vi "Initialize SP.vi"(8 "error in (no error)":errorcluster, 11 "Settings in":refnum<class "Settings.lvclass">) -> (0 "error out":errorcluster, 3 "Settings out":refnum<class "Settings.lvclass">)   [LabVIEW 2023, in "GUI.lvlib" / "Settings.lvlib" / "Settings.lvclass"]
uses:
  Settings.lvclass
  HardwareAbstractionLayer_LVOOP/Database/SQL Public VI/Control/DB Options.ctl
  Settings.lvclass/Settings.ctl
  Reused Code/Subpanels Actor/subpanels/subpanel/subpanel (abstract).lvclass
  HardwareAbstractionLayer_LVOOP/Database/Database.lvclass
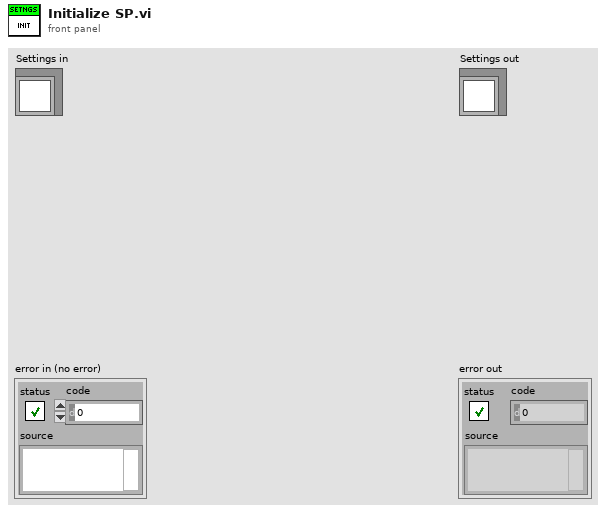
[diagram p1: front panel]
types:
  T1 = typedef "HardwareAbstractionLayer_LVOOP.lvlib/Database.lvclass/DB Options.ctl" = enum16{"Init", "Select Data", "Insert Data", "Update Data", "Delete Data", "Execute Query", "Create Schema", "Create Table", "List Tables", "List Columns", "Close"}
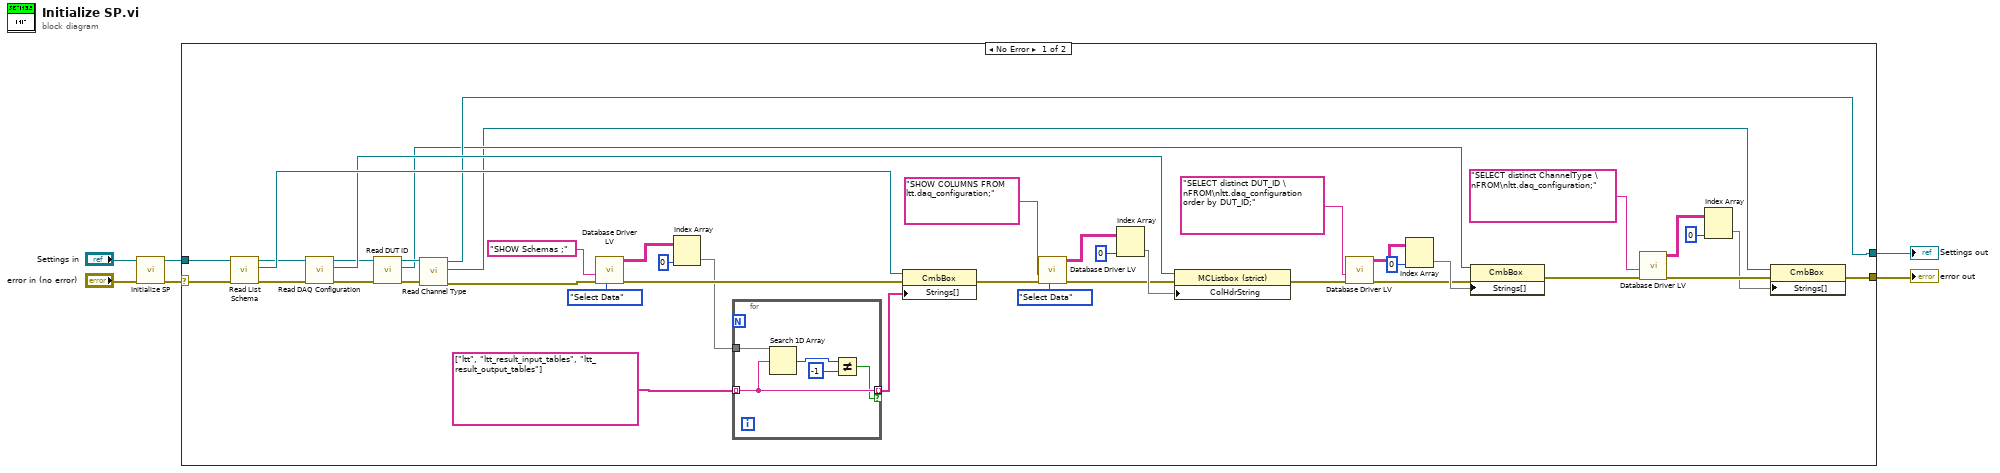
[diagram p0: block diagram]
diagram:
  n1 = call-parent "Initialize SP.vi"("error in (no error)"="error in (no error)", "subpanel (abstract) in"="Settings in") -> ("error out"=w3:errorcluster, "subpanel (abstract) out"=w4:refnum<class "Settings.lvclass">)  [unwired: 8 in]
  n2 = case shown="No Error" w3 {
    selector: w3 -> [w42 w55]
    tunnel: [w19 w55] -> w1
    tunnel: [w12 w54] -> w2
    tunnel: w4 -> [w43 w54]
    frame No Error {
      n3 = call "Read List Schema.vi"("error in (no error)"=w42, "Settings in"=w43) -> ("error out"=w33:errorcluster, "List Schema"=w41:refnum<vi>, "Settings out"=w34:refnum<class "Settings.lvclass">)  [unwired: 7 in]
      n4 = call "Read DAQ Configuration .vi"("error in (no error)"=w33, "Settings in"=w34) -> ("error out"=w17:errorcluster, "DAQ Configuration"=w32:refnum<vi>, "Settings out"=w14:refnum<class "Settings.lvclass">)  [unwired: 7 in]
      n5 = call "Read DUT ID.vi"("error in (no error)"=w17, "Settings in"=w14) -> ("error out"=w16:errorcluster, "DUT ID"=w11:refnum<vi>, "Settings out"=w13:refnum<class "Settings.lvclass">)  [unwired: 7 in]
      n6 = call "Read Channel Type.vi"("error in (no error)"=w16, "Settings in"=w13) -> ("error out"=w15:errorcluster, "Channel Type"=w10:refnum<vi>, "Settings out"=w12:refnum<class "Settings.lvclass">)  [unwired: 7 in]
      n7 = call "Database Driver LV.vi"("Options"=DB_Options."Select Data", "error in"=w15, "SQL query"="SHOW Schemas ;") -> ("error out"=w44:errorcluster, "data"=w46:string[][])  [unwired: 5 in, 2 out]
      n8 = Index Array(array=w46, index (col)=0 ("disabled index (col)")) -> (element=w8:string[])  [unwired: 1 in]
      n9 = for {
        tunnel: string[] ["ltt", "ltt_result_input_tables", "ltt_result_output_tables"] -> [w50] mode=indexing
        tunnel: w8 -> [w51]
        tunnel: [w50] -> w7 mode=indexing if=w49
        n10 = Search 1D Array(1D array=w51, element=w50) -> (index of element=w53:i32)  [unwired: 1 in]
        n11 = Not Equal?(x=w53, y=-1) -> (x != y?=w49:bool)
      }
      n12 = property on="Property Node" class="CmbBox"(reference=w41, error in=w44, "Strings[]"=w7) -> (error out=w35:errorcluster)  [unwired: 1 out]
      n13 = call "Database Driver LV.vi"("Options"=DB_Options."Select Data", "error in"=w35, "SQL query"="SHOW COLUMNS FROM ltt.daq_configuration;") -> ("error out"=w36:errorcluster, "data"=w39:string[][])  [unwired: 5 in, 2 out]
      n14 = Index Array(array=w39, index (col)=0 ("disabled index (col)")) -> (element=w37:string[])  [unwired: 1 in]
      n15 = property on="Property Node" class="MCListbox (strict)"(reference=w32, error in=w36, "ColHdrString"=w37) -> (error out=w25:errorcluster)  [unwired: 1 out]
      n16 = call "Database Driver LV.vi"("error in"=w25, "SQL query"="SELECT distinct DUT_ID \nFROM\nltt.daq_configuration order by DUT_ID;") -> ("error out"=w28:errorcluster, "data"=w30:string[][])  [unwired: 6 in, 2 out]
      n17 = Index Array(array=w30, index (col)=0 ("disabled index (col)")) -> (element=w29:string[])  [unwired: 1 in]
      n18 = property on="Property Node" class="CmbBox"(reference=w11, error in=w28, "Strings[]"=w29) -> (error out=w18:errorcluster)  [unwired: 1 out]
      n19 = call "Database Driver LV.vi"("error in"=w18, "SQL query"="SELECT distinct ChannelType \nFROM\nltt.daq_configuration;") -> ("error out"=w23:errorcluster, "data"=w24:string[][])  [unwired: 6 in, 2 out]
      n20 = Index Array(array=w24, index (col)=0 ("disabled index (col)")) -> (element=w22:string[])  [unwired: 1 in]
      n21 = property on="Property Node" class="CmbBox"(reference=w10, error in=w23, "Strings[]"=w22) -> (error out=w19:errorcluster)  [unwired: 1 out]
    }
    frame Error {
    }
  }
  "error out" <- w1
  "Settings out" <- w2
